vi "DriveExecuteReadSensors.vi"(8 "error in (no error)":errorcluster) -> (0 "error out":errorcluster, 3 "State3":T1={"Speed"=0.0, "Angle"={"VALUE"=0.0, "COS"=1.0, "SIN"=0.0}} {"Angle"."SIN" format="%13.4f"; "Angle"."COS" format="%13.4f"; "Angle"."VALUE" format="%13.4f"}, 5 "State2":T1={"Speed"=0.0, "Angle"={"VALUE"=0.0, "COS"=1.0, "SIN"=0.0}} {"Angle"."SIN" format="%13.4f"; "Angle"."COS" format="%13.4f"; "Angle"."VALUE" format="%13.4f"}, 7 "State1":T1={"Speed"=0.0, "Angle"={"VALUE"=0.0, "COS"=1.0, "SIN"=0.0}} {"Angle"."SIN" format="%13.4f"; "Angle"."COS" format="%13.4f"; "Angle"."VALUE" format="%13.4f"}, 11 "State0":T1={"Speed"=0.0, "Angle"={"VALUE"=0.0, "COS"=1.0, "SIN"=0.0}} {"Angle"."SIN" format="%13.4f"; "Angle"."COS" format="%13.4f"; "Angle"."VALUE" format="%13.4f"})   [LabVIEW 2023]
doc: "Execute for Drie\n\nClosed control loop for drive\n\ninput: \n error in (cluster)\n\noutput:\n error out (cluster)"
uses:
  <vilib>/Rock Robotics/WPI/ThirdParty/JAS_Junk/TrajLib/TypeDef/SWERVE_DRIVE_MODULE_STATE.ctl
  <vilib>/Rock Robotics/WPI/ThirdParty/JAS_Junk/TrajLib/TypeDef/ROTATION2D.ctl
  <vilib>/Rock Robotics/WPI/ThirdParty/JAS_Junk/TrajLib/LinearFilter_LP_BW1_Execute.vi
  <vilib>/Rock Robotics/WPI/ThirdParty/JAS_Junk/TrajLib/SwerveModuleState_New.vi
  <vilib>/Rock Robotics/WPI/ThirdParty/JAS_Junk/TrajLib/VI/SwerveModulePosition_New.vi
  <vilib>/Rock Robotics/WPI/ThirdParty/JAS_Junk/TrajLib/Conv_Feet_Meters.vi
  DriveModuleGetRef.vi
  <vilib>/Rock Robotics/WPI/ThirdParty/JAS_Junk/TrajLib/VI/Conv_Rotations_Degrees.vi
  <vilib>/Rock Robotics/WPI/ThirdParty/JAS_Junk/TrajLib/LinearFilter_ResetToValue.vi
  <vilib>/Rock Robotics/WPI/ThirdParty/JAS_Junk/TrajLib/LinearFilter_Calculate.vi
  <vilib>/Rock Robotics/WPI/ThirdParty/JAS_Junk/TrajLib/Conv_Deg_Radians.vi
  <vilib>/Rock Robotics/WPI/ThirdParty/JAS_Junk/TrajLib/Rotation2d_CreateAngle.vi
  <vilib>/Rock Robotics/WPI/ThirdParty/ADI/ADIS16470/SubVI/ADIS16470 RefNum Registry Get.vi
  DriveGlobal.vi
  <vilib>/Rock Robotics/WPI/ThirdParty/JAS_Junk/TrajLib/LinearFilter_LowPassBW1.vi
  <vilib>/Rock Robotics/WPI/ThirdParty/Phoenix6/Phoenix6_Device_RefNumRegistryGet.vi
  <vilib>/Rock Robotics/WPI/MotorControl/WPI_MotorControlRefNum Registry Get.vi
  <vilib>/Rock Robotics/WPI/ThirdParty/Phoenix6/CANcoderGetters.vi
  <vilib>/Rock Robotics/WPI/ThirdParty/Phoenix6/getters/GetCANcoder_AbsPosition.vi
  <vilib>/Rock Robotics/Network Tables/NT Write Value.vi
  <vilib>/Rock Robotics/Network Tables/NT Write Number.vi
  <vilib>/Rock Robotics/WPI/ThirdParty/REV Robotics/REVLib/SubVI/Public/SPARK Get Encoder Status.vi
  <vilib>/Rock Robotics/WPI/ThirdParty/REV Robotics/REVLib/SubVI/Public/SPARK Get Encoder Status Position.vi
  <vilib>/Rock Robotics/WPI/ThirdParty/REV Robotics/REVLib/SubVI/Public/SPARK Get Encoder Status Velocity.vi
  <vilib>/Rock Robotics/WPI/ThirdParty/JAS_Junk/TrajLib/Trajectory_Library.lvlib
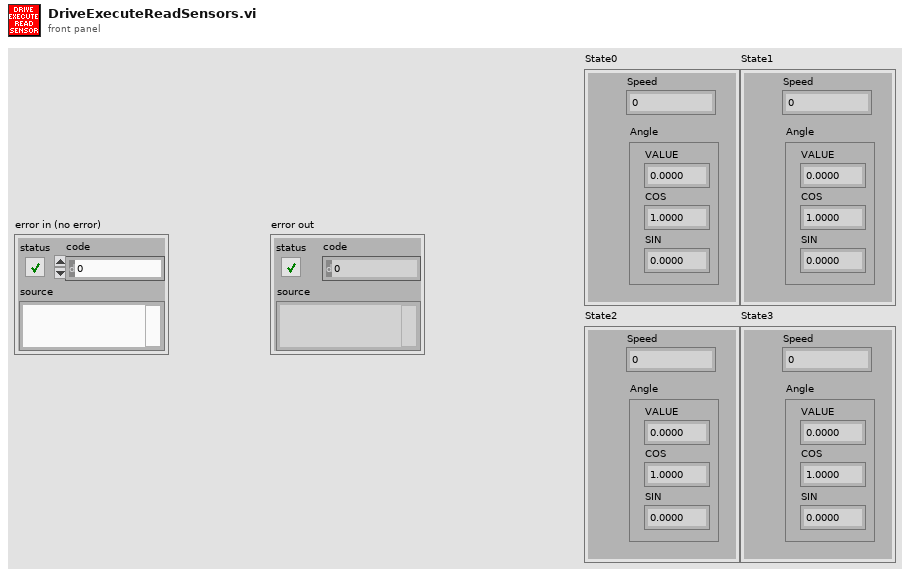
[diagram p1: front panel]
types:
  T1 = typedef "Trajectory_Library.lvlib/SWERVE_DRIVE_MODULE_STATE.ctl" = cluster{"Speed":dbl, "Angle":T2}
  T2 = typedef "Trajectory_Library.lvlib/ROTATION2D.ctl" = cluster{"VALUE":dbl, "COS":dbl, "SIN":dbl}
  T3 = typedef "ADIS16470 Device Reference.ctl" = cluster{"DevStatus":errorcluster, "Hardware Config":T4, "Calibration Complete":refnum<notifier>, "Status Reference":refnum<data-value>, "Data Reference":refnum<data-value>, "Sychronous Process VI":T8, "Cmd FIFO":refnum<k33>, "Source":T9, "Data FIFO":refnum<k33>, "Calibration Time (ms)":u32, "Data Reference":refnum<data-value>}
  T4 = typedef "ADIS16470 Hardware Configuration.ctl" = cluster{"SPI Clock Rate (Hz)":dbl, "IMU SPI Mode (3)":T5, "IMU Reset Pin":T6, "IMU SPI Bus":T7, "IMU Data Ready Pin":T6, "Stall Config":cluster{"Pow2BytesPerRead":u8, "StallTicks":u16, "CsToSclkTicks":u8}}
  T5 = typedef "WPI_SPIMode.ctl" = enum16{"Mode 0 (Clk Idle Low,Sample on Leading)", "Mode 1 (Clk Idle Low,Sample on Trailing)", "Mode 2 (Clk Idle High,Sample on Leading)", "Mode 3 (Clk Idle High,Sample on Trailing)"}
  T6 = typedef "FPGA_DIOChannel.ctl" = enum8{"DIO 0", "DIO 1", "DIO 2", "DIO 3", "DIO 4", "DIO 5", "DIO 6", "DIO 7", "DIO 8", "DIO 9", "DIO MXP 0", "DIO MXP 1", "DIO MXP 2", "DIO MXP 3", "DIO MXP 4", "DIO MXP 5", "DIO MXP 6", "DIO MXP 7", "DIO MXP 8", "DIO MXP 9", "DIO MXP 10", "DIO MXP 11", "DIO MXP 12", "DIO MXP 13", "DIO MXP 14", "DIO MXP 15", "SPI Port CS1", "SPI Port CS2", "SPI Port CS3", "SPI Port MISO", "SPI Port MOSI", "Invalid"}
  T7 = typedef "spi_bus.ctl" = enum16{"SPI On-Board, CS0", "SPI On-Board, CS1", "SPI On-Board, CS2", "SPI On-Board, CS3", "SPI MXP", "Invalid"}
  T8 = typedef "ADIS16470 Process.ctl" = refnum<vi>
  T9 = typedef "FPGA_CounterEncoderSourceConvertionLVSourceType.ctl" = cluster{"DevStatus":errorcluster, "AnalogTriggerMode?":bool, "DigitalMode":cluster{"DIO Channel":T10}, "AnalogTriggerMode":cluster{"AnalogTriggerIndex":T11, "OutputType":T12}}
  T10 = typedef "FPGA_DIODigitalSourceChannel.ctl" = enum8{"DIO 0", "DIO 1", "DIO 2", "DIO 3", "DIO 4", "DIO 5", "DIO 6", "DIO 7", "DIO 8", "DIO 9", "DIO MXP 0", "DIO MXP 1", "DIO MXP 2", "DIO MXP 3", "DIO MXP 4", "DIO MXP 5", "DIO MXP 6", "DIO MXP 7", "DIO MXP 8", "DIO MXP 9", "DIO MXP 10", "DIO MXP 11", "DIO MXP 12", "DIO MXP 13", "DIO MXP 14", "DIO MXP 15", "SPI Port CS1", "SPI Port CS2", "SPI Port CS3", "SPI Port MISO", "SPI Port MOSI", "Disabled"}
  T11 = typedef "FPGA_AnalogTriggerIndex.ctl" = enum8{"Trig 0", "Trig 1", "Trig 2", "Trig 3", "Trig 4", "Trig 5", "Trig 6", "Trig 7", "Invalid"}
  T12 = typedef "FPGA_AnalogTriggerOutType.ctl" = enum16{"InWindow", "TriggerState", "Rising", "Falling"}
  T13 = typedef "Trajectory_Library.lvlib/SWERVE_DRIVE_MODULE_POSITION.ctl" = cluster{"Distance":dbl, "Angle":T2, "P":bool}
  T14 = typedef "ADIS16470 Data.ctl" = cluster{"XAngle":dbl, "YAngle":dbl, "ZAngle":dbl}
  T15 = typedef "ADIS16470 Status.ctl" = cluster{"Calibrated?":bool, "IMU Detected?":bool}
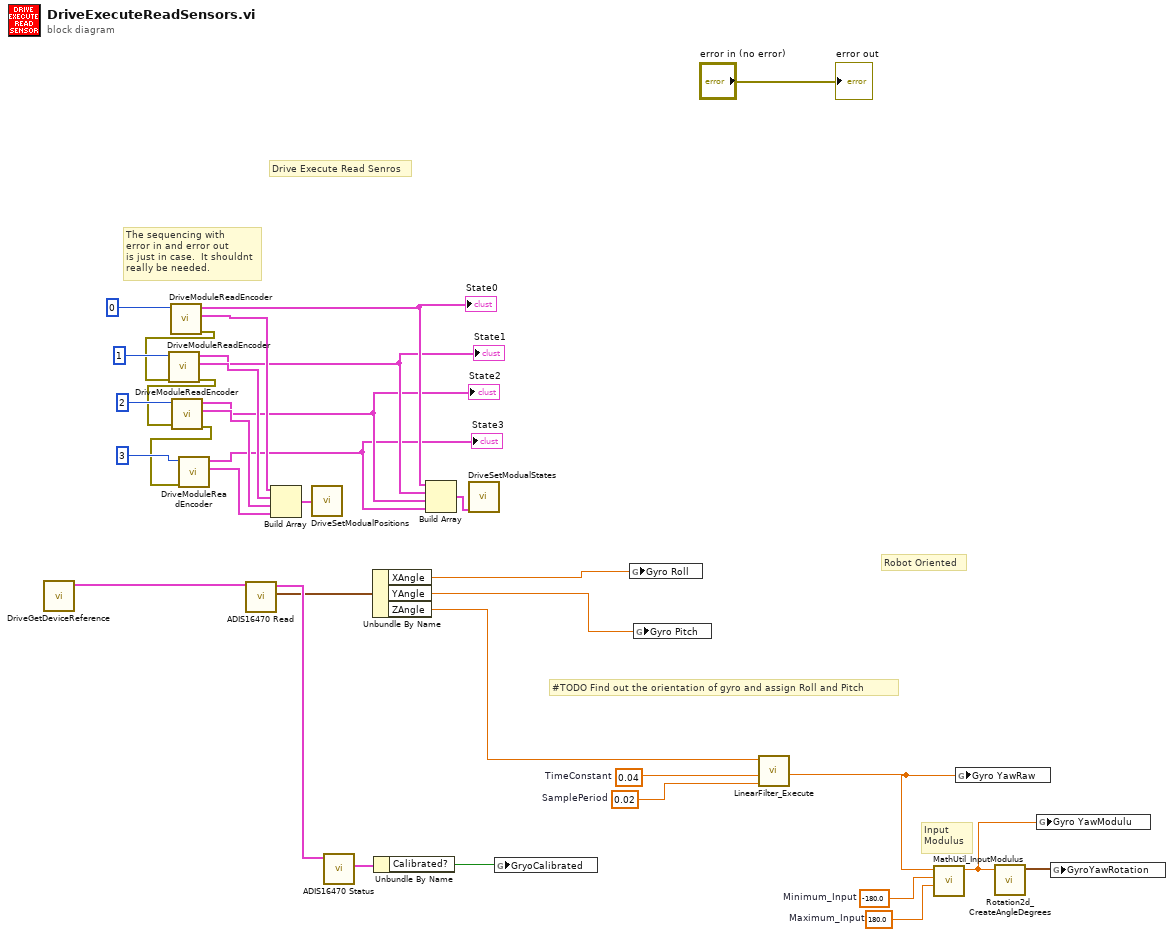
[diagram p0: block diagram]
diagram:
  w11 = -180.0  # Minimum_Input
  w10 = 180.0  # Maximum_Input
  w12 = 0.02  # SamplePeriod
  w13 = 0.04  # TimeConstant
  # "Drive Execute Read Senros"
  # "Input\nModulus"
  # "#TODO Find out the orientation of gyro and assign Roll and Pitch"
  # "Robot Oriented"
  # "The sequencing with\nerror in and error out\nis just in case.  It shouldnt\nreally be needed."
  n1 = call "DriveGetDeviceReference.vi"() -> ("ADIS16470DevRef out"=w18:T3)  [unwired: 11 in]
  n2 = call "DriveModuleReadEncoder.vi"("ModualNamePrefix"=0) -> ("error out"=w21:errorcluster, "SWERVE_DRIVE_MODULE_POSITION"=w27:T13, "SWERVE_DRIVE_MODULE_STATE"=w28:T1)  [unwired: 8 in]
  "State0" <- w28
  n3 = call "DriveModuleReadEncoder.vi"("error in"=w21, "ModualNamePrefix"=1) -> ("error out"=w20:errorcluster, "SWERVE_DRIVE_MODULE_POSITION"=w26:T13, "SWERVE_DRIVE_MODULE_STATE"=w7:T1)  [unwired: 7 in]
  "State1" <- w7
  n4 = call "DriveModuleReadEncoder.vi"("error in"=w20, "ModualNamePrefix"=2) -> ("error out"=w19:errorcluster, "SWERVE_DRIVE_MODULE_POSITION"=w25:T13, "SWERVE_DRIVE_MODULE_STATE"=w6:T1)  [unwired: 7 in]
  "State2" <- w6
  n5 = call "DriveModuleReadEncoder.vi"("error in"=w19, "ModualNamePrefix"=3) -> ("SWERVE_DRIVE_MODULE_POSITION"=w24:T13, "SWERVE_DRIVE_MODULE_STATE"=w5:T1)  [unwired: 7 in, 1 out]
  "State3" <- w5
  n6 = call <vilib>:"ADIS16470 Read.vi"("ADIS16470DevRef"=w18) -> ("ADIS16470 Value"=w14:T14, "ADIS16470DevRef"=w15:T3)  [unwired: 7 in, 2 out]
  n7 = Build Array(w27, w26, w25, w24) -> (w22:T13[])
  n8 = call "DriveSetModualPositions.vi"("Swerve_Drive_Modual_Position"=w22) -> ()  [unwired: 11 in]
  n9 = call <vilib>:"ADIS16470 Status.vi"("ADIS16470DevRef"=w15) -> ("ADIS16470 Status"=w17:T15)  [unwired: 8 in, 2 out]
  n10 = Unbundle By Name(w14) -> ("XAngle"=w1:dbl, "YAngle"=w2:dbl, "ZAngle"=w4:dbl)
  n11 = Unbundle By Name(w17) -> ("Calibrated?"=w16:bool)
  n12 = Build Array(w28, w7, w6, w5) -> (w23:T1[])
  n13 = call "DriveSetModualStates.vi"("Swerve__Drive_Modual_States"=w23) -> ()  [unwired: 11 in]
  n14 = global write "DriveGlobal.vi" "GryoCalibrated"(w16) -> ()
  n15 = global write "DriveGlobal.vi" "Gyro Roll"(w1) -> ()
  n16 = global write "DriveGlobal.vi" "Gyro Pitch"(w2) -> ()
  n17 = call-poly <vilib>:"LinearFilter_Execute.vi"("SamplePeriod"=w12, "TimeConstant"=w13, "Input"=w4) -> ("Output"=w3:dbl)  [unwired: 8 in]
  n18 = call <vilib>:"MathUtil_InputModulus.vi"("Maximum_Input"=w10, "Minimum_Input"=w11, "Input"=w3) -> ("modulus"=w8:dbl)  [unwired: 8 in]
  n19 = global write "DriveGlobal.vi" "Gyro YawRaw"(w3) -> ()
  n20 = call <vilib>:"Rotation2d_CreateAngleDegrees.vi"("Angle_Degrees"=w8) -> ("ROTATION"=w9:T2)  [unwired: 10 in]
  n21 = global write "DriveGlobal.vi" "Gyro YawModulu"(w8) -> ()
  n22 = global write "DriveGlobal.vi" "GyroYawRotation"(w9) -> ()
  "error out" <- "error in (no error)"
